vi "NewFlexUIActorClass.vi"(8 "error in (no error)":errorcluster, 11 "FlexUIActorMaker in":refnum<class "FlexUIActorMaker.lvclass">) -> (0 "error out":errorcluster, 3 "FlexUIActorMaker out":refnum<class "FlexUIActorMaker.lvclass">)   [LabVIEW 2016, in "FlexUIActorMaker.lvlib" / "FlexUIActorMaker.lvclass"]
uses:
  FlexUIActorMaker.lvclass
  FlexUIActorMaker.lvclass/FlexUIActorMaker.ctl
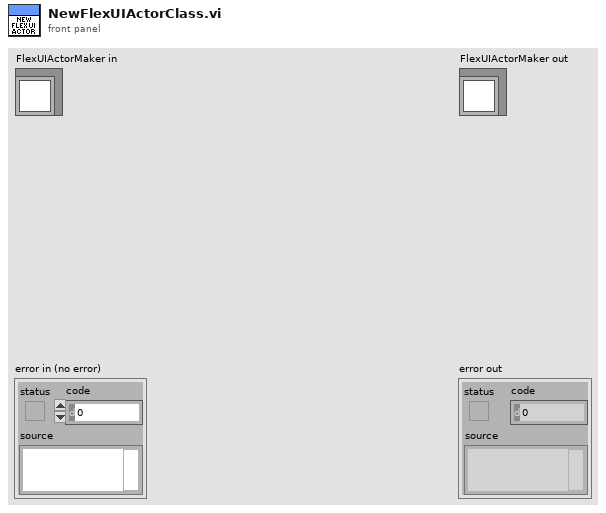
[diagram p1: front panel]
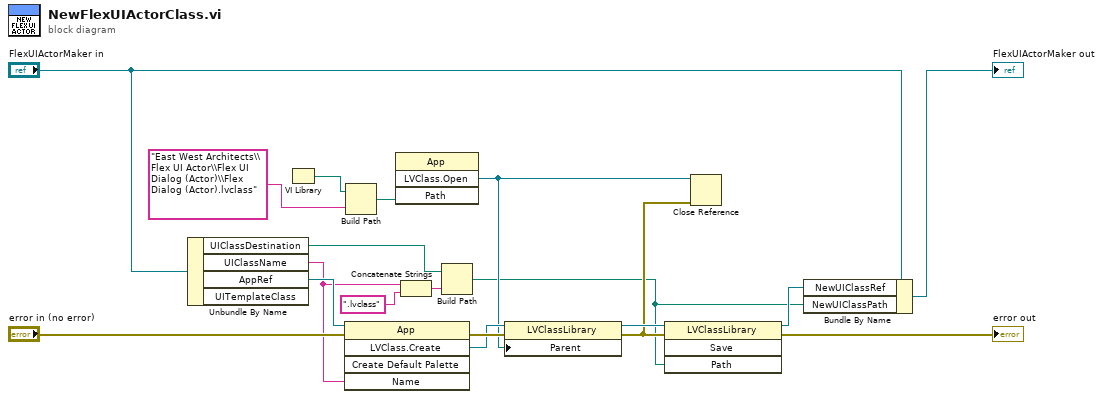
[diagram p0: block diagram]
diagram:
  n1 = Unbundle By Name("FlexUIActorMaker in") -> ("UIClassDestination"=w2:path, "UIClassName"=w5:string, "AppRef"=w13:refnum<vi>)  [unwired: 1 out]
  n2 = VI Library() -> (path=w10:path)
  n3 = invoke class="App" method="LVClass.Create"(reference=w13, error in="error in (no error)", "Name"=w5) -> (error out=w18:errorcluster, "LVClass.Create"=w12:refnum<vi>)  [unwired: 2 in, 3 out]
  n4 = Build Path(base path=w10, name or relative path="East West Architects\\Flex UI Actor\\Flex UI Dialog (Actor)\\Flex Dialog (Actor).lvclass") -> (appended path=w8:path)
  n5 = invoke class="App" method="LVClass.Open"("Path"=w8) -> ("LVClass.Open"=w6:refnum<vi>)  [unwired: 3 in, 3 out]
  n6 = Concatenate Strings(w5, ".lvclass" ("name or relative path")) -> (w3:string)
  n7 = Build Path(base path=w2, name or relative path=w3) -> (appended path=w1:path)
  n8 = property class="LVClassLibrary"(reference=w12, error in=w18, "Parent"=w6) -> (reference out=w11:refnum<vi>, error out=w7:errorcluster)
  n9 = invoke class="LVClassLibrary" method="Save"(reference=w11, error in=w7, "Path"=w1) -> (reference out=w14:refnum<vi>, error out=→"error out":errorcluster)  [unwired: 1 in, 2 out]
  n10 = Close Reference(reference=w6, error in (no error)=w7) -> ()  [unwired: 1 out]
  n11 = Bundle By Name(cluster="FlexUIActorMaker in", "NewUIClassRef"=w14, "NewUIClassPath"=w1) -> (→"FlexUIActorMaker out":refnum<class "FlexUIActorMaker.lvclass">)
